vi "2086组合发送波浪仪.vi"   [LabVIEW 2016, in "数据传输系统-04.lvlib"]
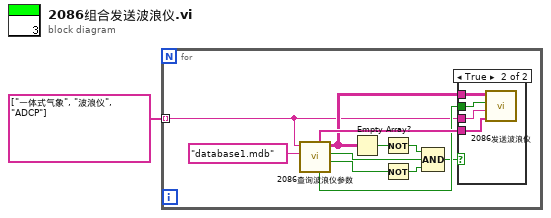
[diagram p0: block diagram]
diagram:
  n1 = for {
    tunnel: string[] ["一体式气象", "波浪仪", "ADCP"] -> [w2] mode=indexing
    n2 = call "2086查询波浪仪参数.vi"("database"="database1.mdb", "table"=w2) -> ("database溢出"=w6:bool, "有数据"=w4:bool, "data"=w9:string[][], "拆分数据"=w8:bool, "columns"=w12:string[])  [unwired: 4 in, 1 out]
    n3 = Empty Array?(array=w9) -> (empty?=w10:bool)
    n4 = Not(x=w10) -> (.not. x?=w11:bool)
    n5 = Not(x=w6) -> (.not. x?=w5:bool)
    n6 = Compound Arithmetic op=AND ("复合运算")(w11, w4, w5) -> (w7:bool)
    n7 = case shown="True" w7 {
      tunnel: w9 -> [_ w16]
      tunnel: w8 -> [_ w15]
      tunnel: w12 -> [_ w14]
      tunnel: w2 -> [_ w13]
      frame False {
      }
      frame True {
        n8 = call "2086发送波浪仪.vi"("columns"=w14, "table"=w13, "拆分数据"=w15, "data"=w16) -> ()  [unwired: 8 in]
      }
    }
  }
